vi "Initialize or Close Instrument Sessions Template.vi"(0 "Semiconductor Module Context":T1, 5 "Operation":enum16{"Initialize", "Close"}(ring), 11 "error in":errorcluster) -> (15 "error out":errorcluster)   [LabVIEW 2023]
uses:
  <vilib>/NI_TestStand_SemiconductorModule/NI_TestStand_Semiconductor_Module.lvlibp/PinMap/General/SemiconductorModuleContext.ctl
  <vilib>/NI_TestStand_SemiconductorModule/NI_TestStand_Semiconductor_Module.lvlibp
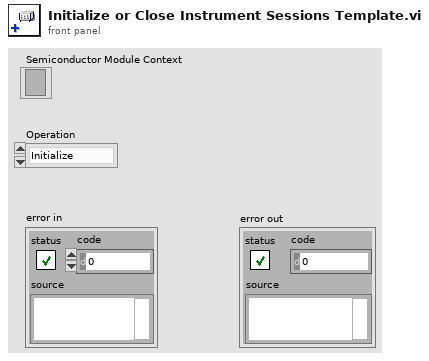
[diagram p1: front panel]
types:
  T1 = typedef "NI_TestStand_Semiconductor_Module.lvlibp/SemiconductorModuleContext.ctl" = refnum<k7>
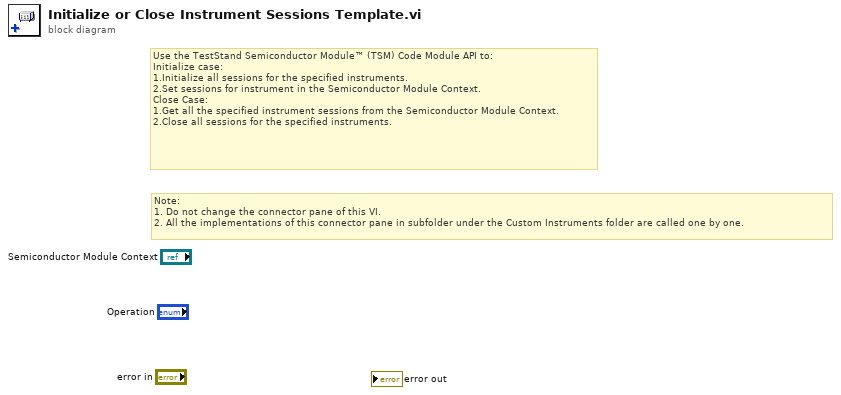
[diagram p0: block diagram]
diagram:
  # "Note: \n1. Do not change the connector pane of this VI.\n2. All the implementations of this connector pane in subfolder under the Custom Instruments folder are called one by one."
  # "Use the TestStand Semiconductor Module™ (TSM) Code Module API to:\nInitialize case:\n1.Initialize all sessions for the specified instruments.\n2.Set sessions for instrument in the Semiconductor Module Context.\nClose Case:\n1.Get all the specified instrument sessions from the Semiconductor Module Context.\n2.Close all sessions for the specified instruments."
